vi "timerRuchuPionowego.vi"(6 "Czynność":T1=enum."działaj", 7 "Pauza":bool, 10 "Czas":dbl, 11 "Wybór komory":T2) -> (3 "Czy czas upłynął?":bool)   [LabVIEW 2014]
uses:
  parametryKomorVIs/WyborKomory.ctl
  poziomyVIs/timerRuchuPoziomegoVIs/Czynnosc.ctl
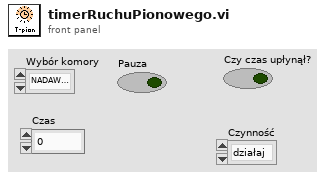
[diagram p1: front panel]
types:
  T1 = typedef "Czynnosc.ctl" = enum16{"reset all", "działaj"}
  T2 = typedef "WyborKomory.ctl" = enum16{"NADAWCZA", "ODBIORCZA"}
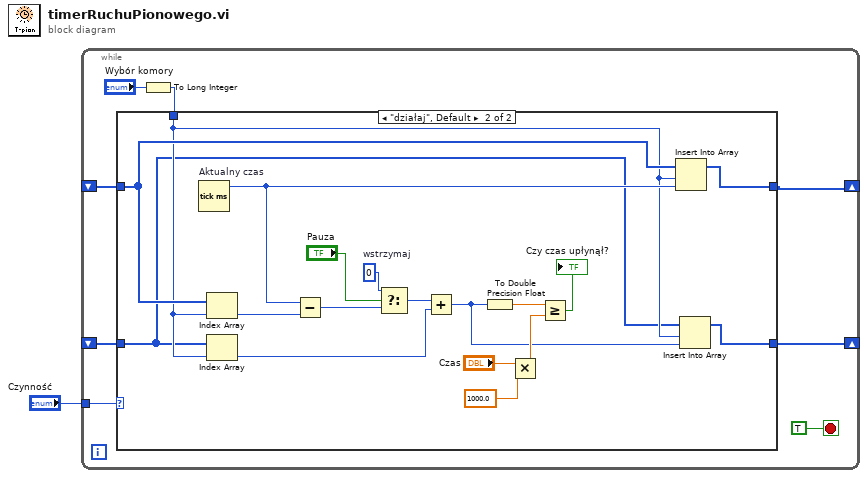
[diagram p0: block diagram]
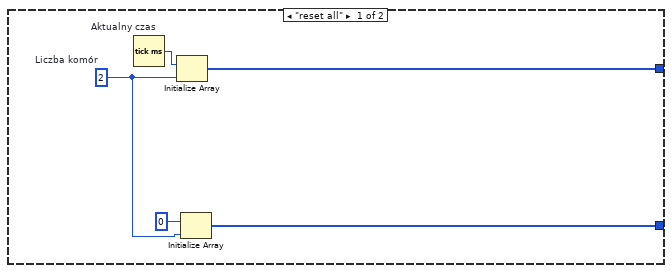
[diagram p2: hidden frame]
diagram:
  n1 = while {
    shift-right: [w3] -> _
    shift-left: _ -> [w6]
    shift-right: [w2] -> _
    shift-left: _ -> [w4]
    tunnel: "Czynność" -> [w8]
    stop <- TRUE stop-if-true
    n2 = To Long Integer(number="Wybór komory") -> (32bit integer=w5:i32)
    n3 = case shown="\"działaj\", Default" w8 {
      tunnel: w6 -> [_ w21]
      tunnel: w5 -> [_ w19]
      tunnel: w4 -> [_ w17]
      tunnel: [w12 w20] -> w3
      tunnel: [w11 w18] -> w2
      frame "reset all" {
        w10 = 2  # Liczba komór
        n4 = Tick Count (ms) "Aktualny czas"() -> (millisecond timer value=w13:u32)
        n5 = Initialize Array(w13, w10) -> (w12:u32[])
        n6 = Initialize Array(u32 0 ("reset"), w10) -> (w11:u32[])
      }
      frame "działaj", Default {
        w31 = u32 0  # wstrzymaj
        n7 = Tick Count (ms) "Aktualny czas"() -> (millisecond timer value=w22:u32)
        n8 = Index Array(array=w21, index=w19) -> (element=w24:u32)
        n9 = Index Array(array=w17, index=w19) -> (element=w23:u32)
        n10 = Subtract(x=w22, y=w24) -> (x-y=w30:u32)
        n11 = Select(t=w31, s="Pauza", f=w30) -> (s? t:f=w32:u32)
        n12 = Add(x=w32, y=w23) -> (x+y=w15:u32)
        n13 = To Double Precision Float(number=w15) -> (double precision float=w25:dbl)
        n14 = Multiply(x="Czas", y=1000.0) -> (x*y=w16:dbl)
        n15 = Greater Or Equal?(x=w25, y=w16) -> (x >= y?=→"Czy czas upłynął?":bool)
        n16 = Insert Into Array(array=w21, index=w19, new element=w22) -> (w20:u32[])
        n17 = Insert Into Array(array=w17, index=w19, new element=w15) -> (w18:u32[])
      }
    }
  }
